vi "XY Graph Sum Selected Plots Event.vi"(8 "Error In":errorcluster, 9 "Add All Plots? (F)":bool, 11 "XYGraph Ref":T1) -> (0 "Error Out":errorcluster, 1 "Message":string, 2 "Sum Plot Name":string, 3 "Added Plot Names":string[](array[string]), 4 "Added Plot Indices":i32[](array[numeric]), 5 "Graph Caption":string)   [LabVIEW 2019, in "XY Graph Add-Ons.lvlib"]
uses:
  XY Graph Add-Ons.lvlib
  XY Graph Refnum.ctl
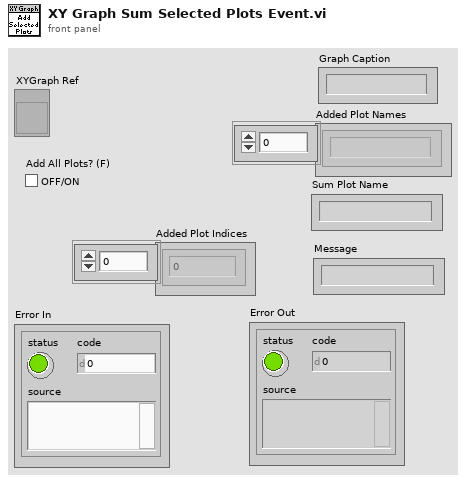
[diagram p1: front panel]
types:
  T1 = typedef "XY Graph Add-Ons.lvlib/XY Graph Refnum.ctl" = refnum<vi>
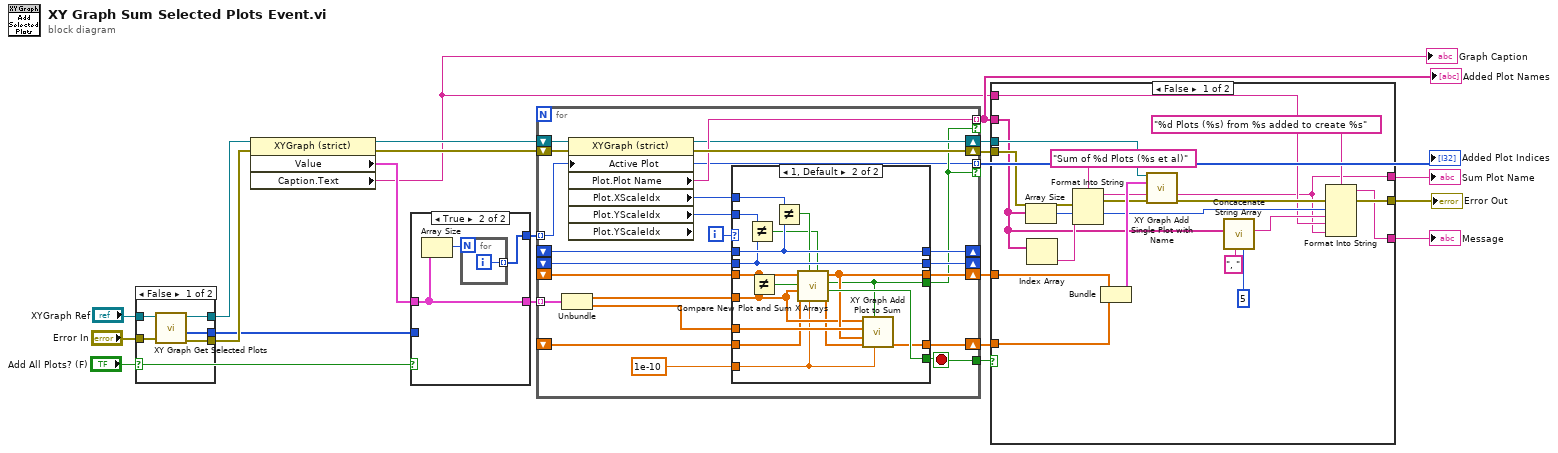
[diagram p0: block diagram]
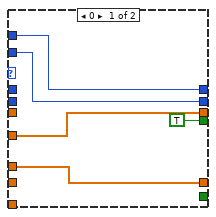
[diagram p3: hidden frame]
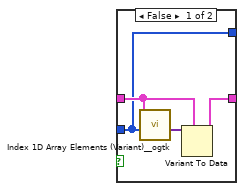
[diagram p4: hidden frame]
diagram:
  n1 = case shown="False" "Add All Plots? (F)" {
    tunnel: "XYGraph Ref" -> [w27 w29]
    tunnel: "Error In" -> [w26 w28]
    tunnel: [w25 w29] -> w20
    tunnel: [w24 _] -> w15
    tunnel: [w23 w28] -> w17
    frame False {
      n2 = call "XY Graph Get Selected Plots.vi"("error in (no error)"=w26, "XYGraph in"=w27) -> ("error out"=w23:errorcluster, "Selected Plots"=w24:i32[], "XYGraph out"=w25:T1)  [unwired: 5 in, 2 out]
    }
    frame True {
    }
  }
  n3 = property class="XYGraph (strict)"(reference=w20, error in=w17) -> (reference out=w18:T1, error out=w14:errorcluster, "Value"=w19:cluster{"X Array":dbl[], "Y Array":dbl[]}[], "Caption.Text"=w1:string)
  "Graph Caption" <- w1
  n4 = case shown="True" "Add All Plots? (F)" {
    tunnel: w19 -> [w32 w36]
    tunnel: [w31 w36] -> w13
    tunnel: w15 -> [w30 _]
    tunnel: [w30 w34] -> w4
    frame False {
      n5 = call <userlib>:"Index 1D Array Elements (Variant)__ogtk.vi"("indices"=w30, "array"=w32) -> ("elements"=w33:variant[])  [unwired: 9 in]
      n6 = Variant To Data(type=w32, Variant=w33) -> (data=w31:cluster{"X Array":dbl[], "Y Array":dbl[]}[])  [unwired: 1 in, 1 out]
    }
    frame True {
      n7 = Array Size(array=w36) -> (size(s)=w35:i32)
      n8 = for {
        N: w35 -> [_]
        tunnel: [w37] -> w34 mode=indexing
        i -> [w37]
      }
    }
  }
  n9 = for {
    tunnel: w13 -> [w60] mode=indexing
    tunnel: [w56] -> w5 mode=indexing if=w41
    tunnel: [w38] -> w7 mode=indexing if=w41
    shift-right: [w53] -> _
    shift-left: _ -> [w48]
    shift-right: [w52] -> _
    shift-left: _ -> [w47]
    shift-right: [w49] -> w12
    shift-left: _ -> [w46]
    shift-right: [w44] -> w11
    shift-left: _ -> [w43]
    shift-right: [w57] -> w10
    shift-left: w14 -> [w58]
    shift-right: [w42] -> w8
    shift-left: w18 -> [w59]
    tunnel: [w40] -> w6
    tunnel: w4 -> [w38] mode=indexing
    i -> [w55]
    stop <- w40 stop-if-true
    n10 = Unbundle(w60) -> ("X Array"=w50:dbl[], "Y Array"=w45:dbl[])
    n11 = property class="XYGraph (strict)" props=["Active Plot", "Plot", "Plot Name", "Plot", "XScaleIdx", "Plot", "YScaleIdx", "Plot", "YScaleIdx"](reference=w59, error in=w58, "Active Plot"=w38) -> (reference out=w42:T1, error out=w57:errorcluster, "Plot.Plot Name"=w56:string, "Plot.XScaleIdx"=w54:u32, "Plot.YScaleIdx"=w51:u32)  [unwired: 1 out]
    n12 = case shown="1, Default" w55 {
      tunnel: w54 -> [w65 w82]
      tunnel: [w65 w81] -> w53
      tunnel: [w64 w79] -> w52
      tunnel: w51 -> [w64 w80]
      tunnel: [w63 w72] -> w49
      tunnel: w50 -> [w63 w69]
      tunnel: w48 -> [_ w81]
      tunnel: w47 -> [_ w79]
      tunnel: w46 -> [_ w75]
      tunnel: w45 -> [w62 w73]
      tunnel: [w62 w71] -> w44
      tunnel: w43 -> [_ w68]
      tunnel: [_ w74] -> w40
      tunnel: [TRUE w70] -> w41
      tunnel: 1e-10 ("epsilon (machine)") -> [_ w66]
      frame 0 {
      }
      frame 1, Default {
        n13 = Not Equal?(x=w80, y=w79) -> (x != y?=w77:bool)
        n14 = Not Equal?(x=w75, y=w69) -> (x != y?=w76:bool)
        n15 = Not Equal?(x=w82, y=w81) -> (x != y?=w78:bool)
        n16 = call "Compare New Plot and Sum X Arrays.vi"("Different Y Scale"=w77, "epsilon (machine)"=w66, "Different X Scale"=w78, "Existing Y Array"=w68, "New X Array in"=w69, "Different X Axis"=w76, "Existing X Array"=w75) -> ("Y Array out"=w67:dbl[], "Cancel"=w74:bool, "Keep Plot"=w70:bool, "X Array out"=w72:dbl[])  [unwired: 1 in]
        n17 = call "XY Graph Add Plot to Sum.vi"("epsilon (machine)"=w66, "Keep Plot"=w70, "Sum Plot Y"=w67, "Sum Plot X"=w72, "New Plot Y"=w73, "New Plot X"=w69) -> ("Sum Plot Y"=w71:dbl[])  [unwired: 5 in]
      }
    }
  }
  "Added Plot Indices" <- w7
  "Added Plot Names" <- w5
  n18 = case shown="False" w6 {
    tunnel: w12 -> [w102 _]
    tunnel: w11 -> [w101 _]
    tunnel: w10 -> [w96 w103]
    tunnel: [w86 w103] -> w9
    tunnel: [w83 _] -> w3
    tunnel: w8 -> [w99 _]
    tunnel: w5 -> [w90 _]
    tunnel: [w85 _] -> w2
    tunnel: w1 -> [w84 _]
    frame False {
      n19 = Array Size(array=w90) -> (size(s)=w89:i32)
      n20 = Index Array(array=w90) -> (element=w94:string)  [unwired: 1 in]
      n21 = Format Into String(format string="Sum of %d Plots (%s et al)" ("initial string"), error in=w96, w89, w94) -> (resulting string=w98:string, error out=w97:errorcluster)  [unwired: 1 in]
      n22 = Bundle("X Array out"=w102, "Sum Plot Y"=w101) -> (w100:cluster{"X Array out":dbl[], "Sum Plot Y":dbl[]})  [unwired: 1 in]
      n23 = call "XY Graph Add Single Plot with Name.vi"("XYGraph Ref in"=w99, "Plot"=w100, "Plot Name (\"Plot\")"=w98, "error in (no error)"=w97) -> ("Plot Name"=w83:string, "error out"=w87:errorcluster)  [unwired: 8 in, 2 out]
      n24 = call "Concacenate String Array.vi"("Max Number of Elements (None: -1)"=5 ("Max Number of Elements (None: 1)"), "Separator (TAB)"=", ", "String Array"=w90) -> ("Formatted String"=w92:string)  [unwired: 8 in]
      n25 = Format Into String(format string="%d Plots (%s) from %s added to create %s", error in=w87, w89, w92, w84, w83) -> (resulting string=w85:string, error out=w86:errorcluster)  [unwired: 1 in]
    }
    frame True {
    }
  }
  "Error Out" <- w9
  "Message" <- w2
  "Sum Plot Name" <- w3
